vi "Initialize.vi"(7 "unit ID":u8=1, 8 "error in":errorcluster, 10 "baudRate (9600)":u32=9600, 11 "VISA resource name":refnum<visa-resource-name>) -> (0 "error out":errorcluster, 3 "serial master instance":refnum<class "Modbus Master.lvclass">)   [LabVIEW 2025, in "Hanmatek HM310T.lvlib"]
uses:
  <vilib>/NI/Modbus Library/API/Master/Modbus Master.lvclass
  f8f31601-b21c-4c8d-ab26-724c93e45244.vi
  <vilib>/NI/Modbus Library/API/Wrapper/Create Serial Master.vi
  <instrlib>/Hanmatek HM310T/Hanmatek HM310T.lvlib
  <vilib>/NI/Modbus Library/API/Wrapper/API Main.lvlib
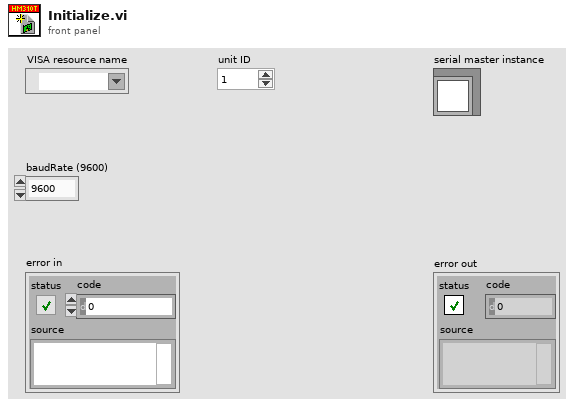
[diagram p1: front panel]
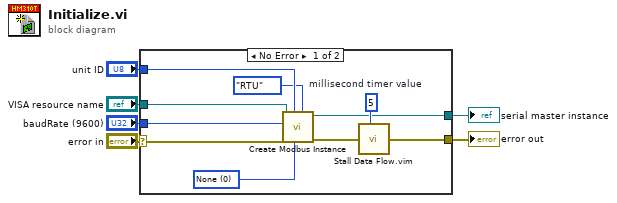
[diagram p0: block diagram]
diagram:
  n1 = case shown="No Error" "error in" {
    selector: "error in" -> [w9 w17]
    tunnel: [w16 w17] -> w6
    tunnel: "baudRate (9600)" -> [w13 _]
    tunnel: "VISA resource name" -> [w12 _]
    tunnel: [w11 _] -> w3
    tunnel: "unit ID" -> [w10 _]
    frame No Error {
      w8 = u16 0 items=["None", "Odd", "Even", "Mark", "Space"] ("parity (even)")
      w14 = u32 5  # millisecond timer value
      n2 = call-poly <vilib>:"Create Modbus Instance.vi"("serial type"=enum16{"RTU", "ASCII"}."RTU", "parity (even)"=w8, "unit ID"=w10, "error in"=w9, "baud rate"=w13, "VISA resource name"=w12) -> ("error out"=w15:errorcluster, "serial master instance"=w11:refnum<class "Modbus Master.lvclass">)  [unwired: 4 in]
      n3 = call "Stall Data Flow.vim"("value in"=w15, "milliseconds to wait"=w14) -> ("value out"=w16:errorcluster)  [unwired: 1 out]
    }
    frame Error {
    }
  }
  "error out" <- w6
  "serial master instance" <- w3
